vi "Read History.vi"(8 "error in (no error)":errorcluster, 11 "Fault Monitor in":refnum<class "Fault Monitor.lvclass">) -> (0 "error out":errorcluster, 3 "Fault Monitor out":refnum<class "Fault Monitor.lvclass">)   [LabVIEW 2023, in "Fault Monitor.lvlib" / "Fault Monitor.lvclass"]
uses:
  Library/Fault Monitor.lvclass
  Library/Fault Monitor.lvclass/Fault Monitor.ctl
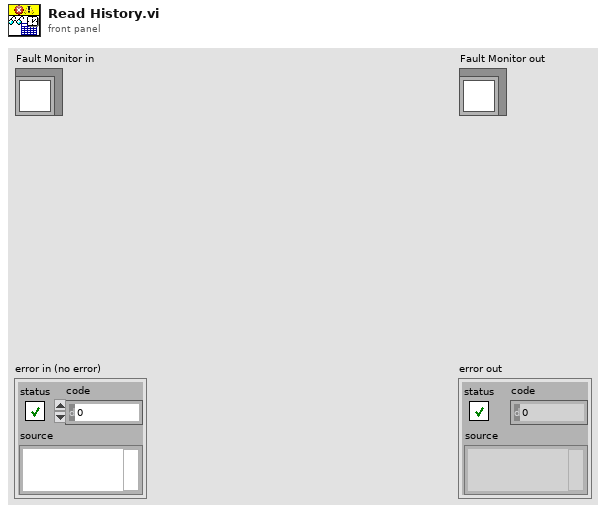
[diagram p1: front panel]
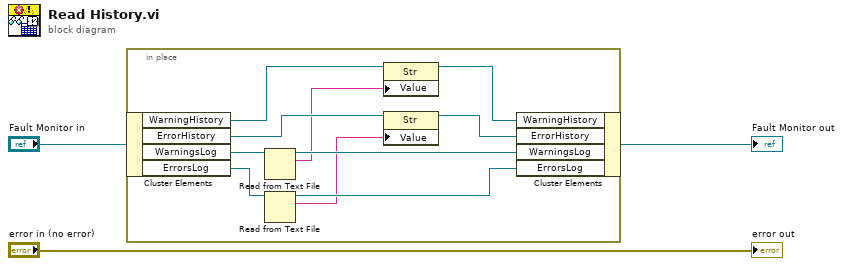
[diagram p0: block diagram]
diagram:
  n1 = in-place {
    n2 = in-place-cluster #1("Fault Monitor in") -> ("WarningHistory"=w9:refnum<vi>, "ErrorHistory"=w8:refnum<vi>, "WarningsLog"=w13:refnum<file>, "ErrorsLog"=w12:refnum<file>)
    n3 = Read from Text File(file (use dialog)=w13) -> (refnum out=w11:refnum<file>, text=w5:string)  [unwired: 3 in, 2 out]
    n4 = Read from Text File(file (use dialog)=w12) -> (refnum out=w10:refnum<file>, text=w4:string)  [unwired: 3 in, 2 out]
    n5 = property class="Str"(reference=w9, "Value"=w5) -> (reference out=w6:refnum<vi>)  [unwired: 1 in, 1 out]
    n6 = property class="Str"(reference=w8, "Value"=w4) -> (reference out=w7:refnum<vi>)  [unwired: 1 in, 1 out]
    n7 = in-place-cluster #1("WarningHistory"=w6, "ErrorHistory"=w7, "WarningsLog"=w11, "ErrorsLog"=w10) -> (→"Fault Monitor out":refnum<class "Fault Monitor.lvclass">)
  }
  "error out" <- "error in (no error)"
